vi "Max Read Array.vi"(8 "error in":errorcluster, 11 "Max Flow Limit in":refnum<class "Flow Limit.lvclass">) -> (0 "error out":errorcluster, 1 "Changed or First Call?":bool, 2 "Flow Max SP":dbl[](array[numeric]), 3 "Max Flow Limit out":refnum<class "Flow Limit.lvclass">)   [LabVIEW 2023, in "Flow Limit.lvclass"]
uses:
  Flow Limit.lvclass
  Parents/Limit/Limit.lvclass
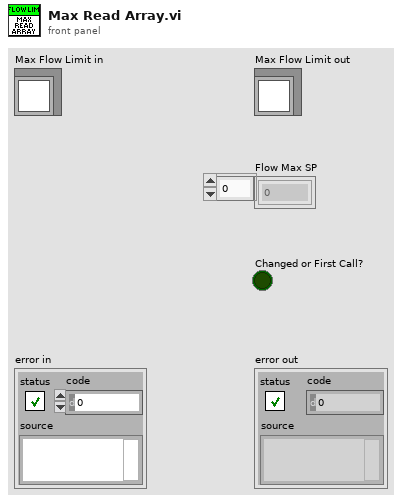
[diagram p1: front panel]
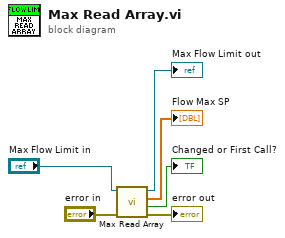
[diagram p0: block diagram]
diagram:
  n1 = call-parent "Max Read Array.vi"("error in"="error in", "Max Limit in"="Max Flow Limit in") -> ("error out"=→"error out":errorcluster, "Changed or First Call?"=→"Changed or First Call?":bool, "Current Max SP"=→"Flow Max SP":dbl[], "Max Limit out"=→"Max Flow Limit out":refnum<class "Flow Limit.lvclass">)  [unwired: 6 in]
